vi "Battery_Create.vi"(0 "reference in":refnum<class "Battery.lvclass">, 1 "Rated Capacity (AH)":dbl=1.0, 2 "Discharge Current (A)":dbl=1.0, 3 "Charge Current (A)":dbl=1.0, 4 "Discharge Cutoff (V)":dbl=2.8, 5 "Error In":errorcluster, 6 "Starting Voltage (V)":dbl=3.5, 7 "Internal Resistance (0.02 Ohm)":dbl=0.02, 8 "Nominal Voltage (V)":dbl=3.7) -> (14 "reference out":refnum<class "Battery.lvclass">, 15 "ProcessViRef":refnum<vi>, 19 "Error Out":errorcluster)   [LabVIEW 2023, in "Battery.lvclass"]
uses:
  Battery.lvclass
  Battery.lvclass/Battery.ctl
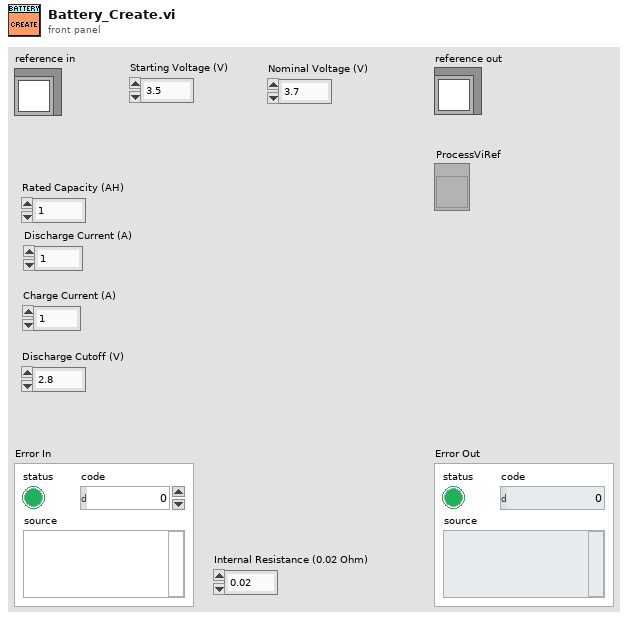
[diagram p1: front panel]
types:
  T1 = enum16{"Disconnected", "Charging", "Discharging"}
  T2 = typedef "Battery.lvclass/ObjectAttributes.ctl" = cluster{"Mode":enum16{"Disconnected", "Charging", "Discharging"}, "Discharge Switch":bool, "Cell Voltage (V)":dbl, "Cell Current (A)":dbl, "SoC (%)":dbl, "Nominal Voltage (V)":dbl, "Model Index":i32}
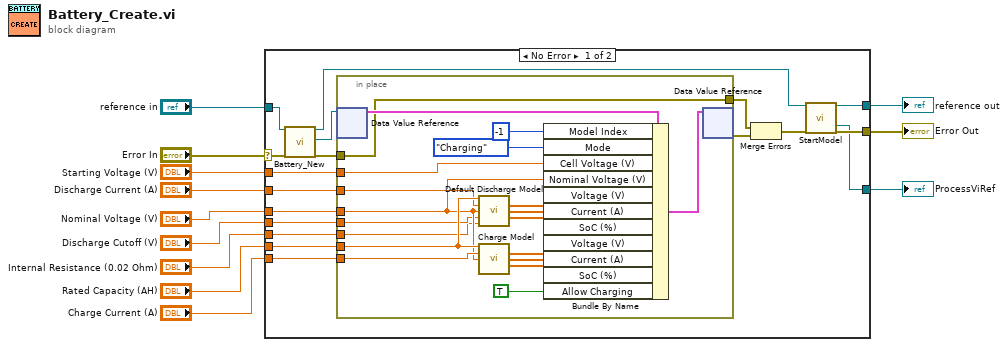
[diagram p0: block diagram]
diagram:
  n1 = case shown="No Error" "Error In" {
    selector: "Error In" -> [w29 w51]
    tunnel: [w21 w51] -> w11
    tunnel: "reference in" -> [w30 w50]
    tunnel: [w23 w50] -> w9
    tunnel: "Rated Capacity (AH)" -> [w18 _]
    tunnel: "Discharge Current (A)" -> [w16 _]
    tunnel: "Charge Current (A)" -> [w17 _]
    tunnel: "Nominal Voltage (V)" -> [w20 _]
    tunnel: "Internal Resistance (0.02 Ohm)" -> [w14 _]
    tunnel: "Discharge Cutoff (V)" -> [w15 _]
    tunnel: "Starting Voltage (V)" -> [w19 _]
    tunnel: [w13 _] -> w1
    frame No Error {
      n2 = call "Battery_New.vi"("reference in"=w30, "Error In"=w29) -> ("reference out"=w24:refnum<class "Battery.lvclass">, "DVRRefOut"=w27:refnum<data-value>, "Error Out"=w26:errorcluster)  [unwired: 14 in, 1 out]
      n3 = in-place {
        in-place-border: w26 -> [w47]
        in-place-border: [w47] -> w25
        in-place-border: w20 -> [w40]
        in-place-border: w19 -> [w44]
        in-place-border: w18 -> [w42]
        in-place-border: w17 -> [w43]
        in-place-border: w16 -> [w41]
        in-place-border: w15 -> [w39]
        in-place-border: w14 -> [w38]
        n4 = in-place-dvr #1(w27) -> (w48:T2)  [unwired: 1 out]
        n5 = call "Default Discharge Model.vi"("Rated Capacity (AH)"=w42, "Discharge Current (A)"=w41, "Cell Voltage (V)"=w40, "Cutoff Voltage (V)"=w39, "Internal Resistance (0.02 Ohm)"=w38) -> ("Cell Voltage (V)"=w34:dbl[], "Cell Current (A)"=w33:dbl[], "SoC (%)"=w32:dbl[])  [unwired: 8 in]
        n6 = call "Charge Model.vi"("Rated Capacity (AH)"=w42, "Charge Current (A)"=w43, "Cell Voltage (V)"=w40) -> ("Cell Voltage (V)"=w37:dbl[], "Cell Current (A)"=w36:dbl[], "SoC (%)"=w35:dbl[])  [unwired: 10 in]
        n7 = Bundle By Name(cluster=w48, "Model Index"=-1, "Mode"=T1."Charging", "Cell Voltage (V)"=w44, "Nominal Voltage (V)"=w40, "Voltage (V)"=w34, "Current (A)"=w33, "SoC (%)"=w32, "Voltage (V)"=w37, "Current (A)"=w36, "SoC (%)"=w35, "Allow Charging"=TRUE) -> (w49:T2)
        n8 = in-place-dvr #1(w49) -> (w28:errorcluster)  [unwired: 1 out]
      }
      n9 = Merge Errors(w25, w28) -> (w22:errorcluster)
      n10 = call "StartModel.vi"("reference in"=w24, "Error In"=w22) -> ("reference out"=w23:refnum<class "Battery.lvclass">, "ProcessViRef"=w13:refnum<vi>, "Error Out"=w21:errorcluster)  [unwired: 13 in, 2 out]
    }
    frame Error {
      # "VI-TechBaseTemplate_Simple_6x8x6"
    }
  }
  "Error Out" <- w11
  "reference out" <- w9
  "ProcessViRef" <- w1
